vi "matrici_v31.vi"() -> ()   [LabVIEW 2009]
uses:
  <vilib>/Analysis/Matrix/Datatypes/ComplexMatrix.ctl
  <vilib>/Analysis/Matrix/NI_Matrix.lvlib
panel:
  in  "stop":bool
  out "Complex Matrix":T1=[[20.346672630653416+53.85940377630152i, 96.028134804551+21.918836536570822i, 20.66647244731503+54.83786879323276i], [98.87921293213536+40.90568843678915i, 35.888357976791774+56.52820368000566i, 17.306282315549115+7.648351339847381i], [99.4135818272078+34.93250306063946i, 82.88847066391338+71.22601142956702i, 67.38944241247826+52.54366844889189i], [14.039689947692002+79.33060951656319i, 34.55202918251066+67.10730058563274i, 43.149466876709084+30.308385792195345i], [73.8986175169019+82.38713511067755i, 80.45114809724807+39.6020359456873i, 97.27537671676751+92.87466973467306i]]
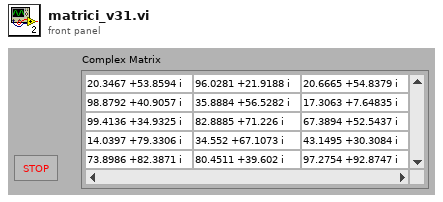
[diagram p1: front panel]
types:
  T1 = typedef "NI_Matrix.lvlib/ComplexMatrix.ctl" = cdb[][]
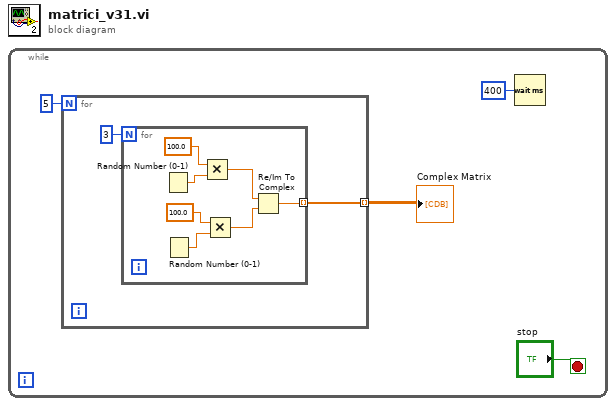
[diagram p0: block diagram]
diagram:
  n1 = while {
    stop <- "stop" stop-if-true
    n2 = for {
      N: 5 -> [_]
      tunnel: [w5] -> w3 mode=indexing
      n3 = for {
        N: 3 -> [_]
        tunnel: [w13] -> w5 mode=indexing
        n4 = Random Number (0-1)() -> (number: 0 to 1=w12:dbl)
        n5 = Random Number (0-1)() -> (number: 0 to 1=w11:dbl)
        n6 = Multiply(x=100.0, y=w12) -> (x*y=w8:dbl)
        n7 = Multiply(x=100.0, y=w11) -> (x*y=w7:dbl)
        n8 = Re/Im To Complex(1:w7, 2:w8) -> (0:w13:cdb)
      }
    }
    "Complex Matrix" <- w3
    n9 = Wait (ms)(milliseconds to wait=u32 400) -> ()  [unwired: 1 out]
  }
